vi "Find Hardware.vi"() -> (0 "error out":errorcluster, 1 "Product Category":i32[](array[ring]) items=["M Series DAQ"=14643, "X Series DAQ"=15858, "E Series DAQ"=14642, "S Series DAQ"=14644, "B Series DAQ"=14662, "SC Series DAQ"=14645, "USB DAQ"=14646, "AO Series"=14647, "Digital I/O"=14648, "TIO Series"=14661, "Dynamic Signal Acquisition"=14649, "Switches"=14650, "CompactDAQ Chassis"=14658, "CompactRIO Chassis"=16144, "C Series Module"=14659, "SCXI Module"=14660, "SCC Connector Block"=14704, "SCC Module"=14705, "NI ELVIS"=14755, "Network DAQ"=14829, "SC Express"=15886, "FieldDAQ"=16151, "TestScale Chassis"=16180, "TestScale Module"=16181, "mioDAQ"=16182, "Unknown"=12588], 2 "DevNames":tag[](array[tag]), 3 "Device Type":string[](array[string]))   [LabVIEW 2025, in "USB IO.lvlib" / "USB IO.lvclass"]
uses:
  USB IO.lvclass
  USB IO.lvclass/USB IO.ctl
  <resource>/objmgr/daqmx.rc
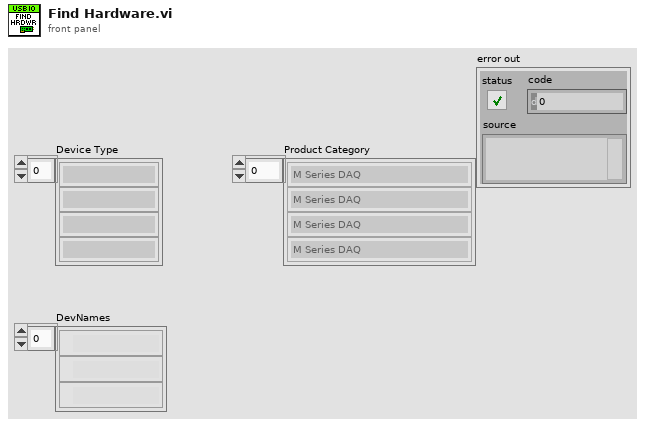
[diagram p1: front panel]
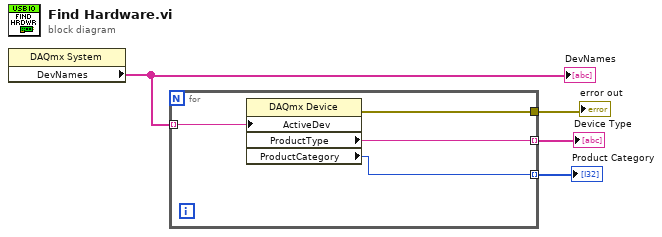
[diagram p0: block diagram]
diagram:
  n1 = property class="DAQmx System"() -> ("DevNames"=w3:tag[])  [unwired: 2 in, 2 out]
  "DevNames" <- w3
  n2 = for {
    tunnel: w3 -> [w8] mode=indexing
    tunnel: [w7] -> w4 mode=indexing
    tunnel: [w6] -> w2 mode=indexing
    tunnel: [w5] -> w1
    n3 = property class="DAQmx Device"("ActiveDev"=w8) -> (error out=w5:errorcluster, "ProductType"=w7:string, "ProductCategory"=w6:i32)  [unwired: 2 in, 1 out]
  }
  "Device Type" <- w4
  "Product Category" <- w2
  "error out" <- w1
